vi "SimpleGit-Status.vi"(11 "path":path) -> ()   [LabVIEW 2017]
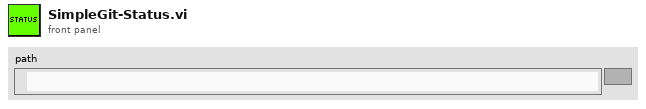
[diagram p1: front panel]
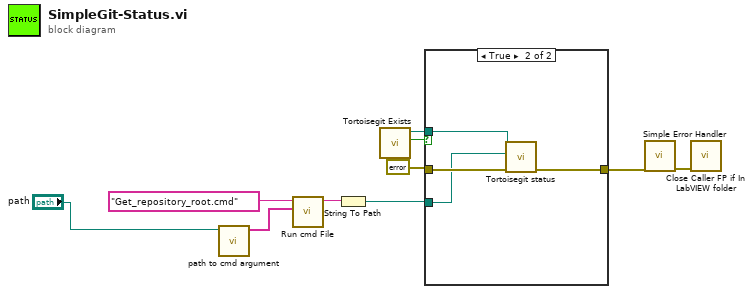
[diagram p0: block diagram]
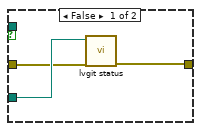
[diagram p2: hidden frame]
diagram:
  n1 = call "path to cmd argument.vi"("path"="path") -> ("Array"=w5:string[])  [unwired: 10 in]
  n2 = call "Run cmd File.vi"("args"=w5, "name or relative path"="Get_repository_root.cmd") -> ("standard output"=w3:string)  [unwired: 7 in, 2 out]
  n3 = String To Path(string=w3) -> (path=w2:path)
  n4 = call "Tortoisegit Exists.vi"() -> ("file or folder exists?"=w8:bool, "TortoiseGitProc.exe"=w7:path)  [unwired: 10 in]
  n5 = case shown="True" w8 {
    tunnel: errorcluster {"status"=FALSE, "code"=0, "source"=""} ("error in") -> [w12 w17]
    tunnel: w7 -> [_ w15]
    tunnel: w2 -> [w13 w16]
    tunnel: [w11 w14] -> w6
    frame False {
      n6 = call "lvgit status.vi"("error in"=w12, "path"=w13) -> ("error out"=w11:errorcluster)  [unwired: 9 in]
    }
    frame True {
      n7 = call "Tortoisegit status.vi"("error in (no error)"=w17, "path"=w16, "TortoiseGitProc.exe"=w15) -> ("error out"=w14:errorcluster)  [unwired: 8 in]
    }
  }
  n8 = call <vilib>:"Simple Error Handler.vi"("error in (no error)"=w6) -> ("error out"=w9:errorcluster)  [unwired: 4 in, 4 out]
  n9 = call "Close Caller FP if In LabVIEW folder.vi"("error in (no error)"=w9) -> ()  [unwired: 10 in, 1 out]
